vi "Kursory do listbox.vi"(9 "CrsrList":T1, 11 "error in (no error)":errorcluster) -> (1 "Cursors list":string[][](array[string]), 3 "error out":errorcluster)   [LabVIEW 2013]
doc: "Konwertuje listê kursorów do listy\ntypu multikolumn list box"
uses:
  <vilib>/Utility/miscctls.llb/LVCursorListTypeDef.ctl
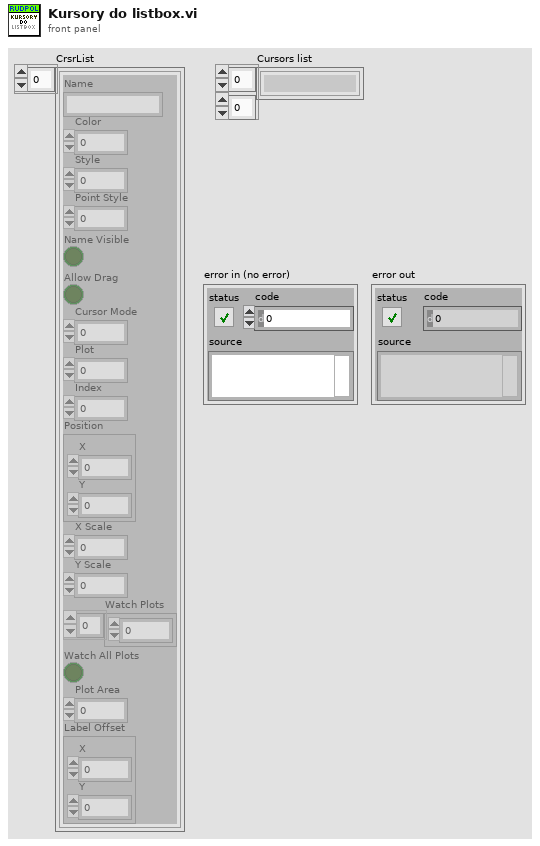
[diagram p1: front panel]
types:
  T1 = typedef "LVCursorListTypeDef.ctl" = cluster{"Name":string, "Color":u32, "Style":u8, "Point Style":u8, "Name Visible":bool, "Allow Drag":bool, "Cursor Mode":u32, "Plot":i32, "Index":i32, "Position":cluster{"X":dbl, "Y":dbl}, "X Scale":u32, "Y Scale":u32, "Watch Plots":i32[], "Watch All Plots":bool, "Plot Area":i32, "Label Offset":cluster{"X":dbl, "Y":dbl}}[]
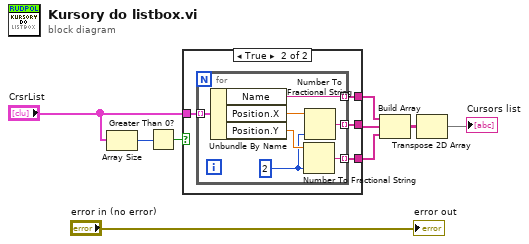
[diagram p0: block diagram]
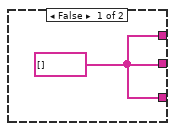
[diagram p2: hidden frame]
diagram:
  n1 = Array Size(array="CrsrList") -> (size(s)=w3:i32)
  n2 = Greater Than 0?(x=w3) -> (x > 0?=w4:bool)
  n3 = case shown="True" w4 {
    tunnel: "CrsrList" -> [_ w14]
    tunnel: [w10 w13] -> w5
    tunnel: [w10 w12] -> w6
    tunnel: [w10 w11] -> w7
    frame False {
      w10 = string[] []
    }
    frame True {
      n4 = for {
        tunnel: w14 -> [w21] mode=indexing
        tunnel: [w20] -> w13 mode=indexing
        tunnel: [w18] -> w12 mode=indexing
        tunnel: [w15] -> w11 mode=indexing
        w16 = i16 2 ("precision (6)")
        n5 = Unbundle By Name(w21) -> ("Name"=w20:string, "Position.X"=w19:dbl, "Position.Y"=w17:dbl)
        n6 = Number To Fractional String(number=w17, precision (6)=w16) -> (F-format string=w15:string)  [unwired: 2 in]
        n7 = Number To Fractional String(number=w19, precision (6)=w16) -> (F-format string=w18:string)  [unwired: 2 in]
      }
    }
  }
  n8 = Build Array(w5, w6, w7) -> (w8:string[][])
  n9 = Transpose 2D Array(2D array=w8) -> (transposed array=→"Cursors list":string[][])
  "error out" <- "error in (no error)"
